vi "Command_Joints.vi"(4 "Mode":T2(ring), 6 "error in":errorcluster, 7 "Arm Angles (degrees)":dbl[](array[numeric]), 9 "Side":T3) -> (0 "error out":errorcluster, 3 "JointCommand":T1={"Mode"=enum."Position", "Arm Angles"=[], "Angle Names"=["_s0", "_s1", "_e0", "_e1", "_w0", "_w1", "_w2"]})   [LabVIEW 2013]
uses:
  ROS/Code/SubVIs/BaxterSide.ctl
  ROS/RosMessages/Clusters/JointCommand.ctl
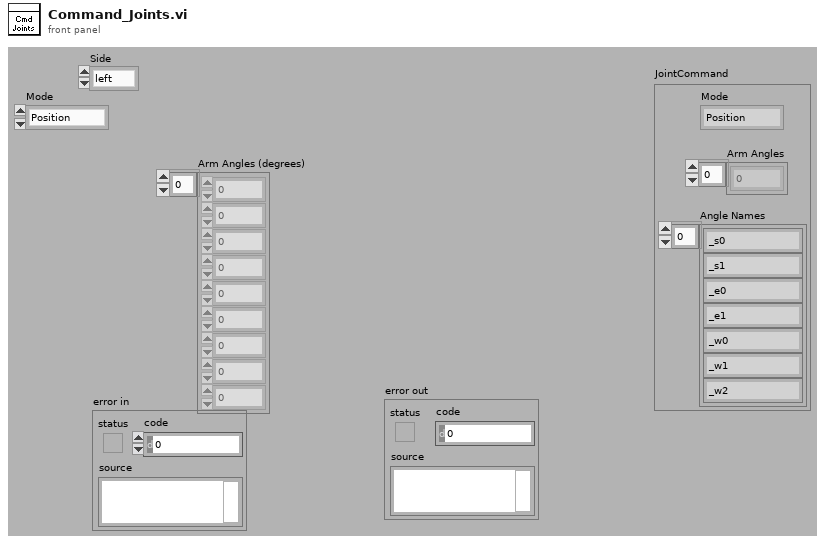
[diagram p1: front panel]
types:
  T1 = typedef "JointCommand.ctl" = cluster{"Mode":enum32{"", "Position", "Velocity", "Effort"}, "Arm Angles":dbl[], "Angle Names":string[]}
  T2 = enum32{"Position", "Velocity", "Effort", "Pause", "Repeat", "End"}
  T3 = typedef "BaxterSide.ctl" = enum16{"left", "right"}
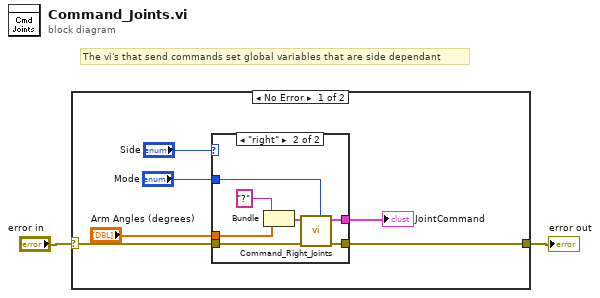
[diagram p0: block diagram]
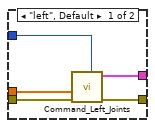
[diagram p2: hidden frame]
diagram:
  # "The vi's that send commands set global variables that are side dependant"
  n1 = case shown="No Error" "error in" {
    selector: "error in" -> [w4 w21]
    tunnel: [w3 w21] -> w2
    frame No Error {
      n2 = case shown="\"right\"" "Side" {
        tunnel: "Mode" -> [w12 w20]
        tunnel: "Arm Angles (degrees)" -> [w11 w15]
        tunnel: [w13 w19] -> w5
        tunnel: w4 -> [w10 w18]
        tunnel: [w9 w17] -> w3
        frame "left", Default {
          n3 = call "Command_Left_Joints.vi"("Mode"=w12, "error in"=w10, 7:w11) -> ("error out"=w9:errorcluster, "JointCommand"=w13:T1)  [unwired: 5 in]
        }
        frame "right" {
          n4 = Bundle("?", "Arm Angles (degrees)"=w15) -> (w16:cluster{string, "Arm Angles (degrees)":dbl[]})  [unwired: 1 in]
          n5 = call "Command_Right_Joints.vi"("Mode"=w20, "error in"=w18, "Goal"=w16) -> ("error out"=w17:errorcluster, "JointCommand"=w19:T1)  [unwired: 5 in]
        }
      }
      "JointCommand" <- w5
    }
    frame Error {
    }
  }
  "error out" <- w2
